vi "merFISH_read_next_task.vi"(3 "error in":errorcluster, 5 "merFISH parameters":T2) -> (0 "error out":errorcluster, 1 "task":T1, 2 "merFISH parameters":T2)   [LabVIEW 2015]
uses:
  CONTROLS/Q_main_element.ctl
  GLOBAL/Global_ABORT.vi
panel:
  out "Instruction":T3(ring)
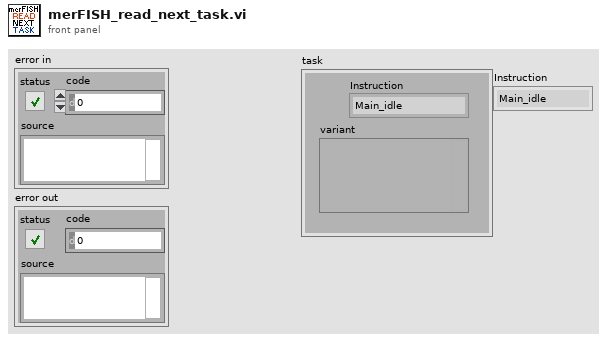
[diagram p1: front panel]
types:
  T1 = typedef "Q_main_element.ctl" = cluster{"variant":variant, "Instruction":enum16{"Main_idle", "Main_initialize", "Main_initialize_TDMS", "Main_initialize_Queue", "Main_error", "Main_DAQ_initialization_results", "Main_ASI_initialization_results", "Main_Piezo_initialization_results", "Main_Valve_initialization_results", "Main_Pump_initialization_results", "Main_CAMERA_initialization_results", "Main_DAQ_error", "Main_ASI_error", "Main_Piezo_error", "Main_CAMERA_error", "Main_Valve_error", "Main_Pump_error", "Main_start_acquiring", "Main_not_acquiring", "Main_acquiring", "Main_stop_acquiring", "Main_change_exposure", "Main_change_z_scan_parameters", "Main_define_ROI", "Main_read_kinetic_time", "Main_cooler", "Main_read_temperature", "Main_save_XY", "Main_load_XY", "Main_discard_XY", "Main_move_to_XY", "Main_measure_QPD", "Main_autofocus_calibration", "Main_save_PID", "Main_change_H_valve_position", "Main_two_way_valve", "Main_save_movie", "Main_init_single_scan", "Main_single_scan", "Main_stop_single_scan", "Main_merFISH_illumination_parameters", "Main_merFISH_buffer_probe_list", "Main_merFISH_injections_procedure", "Main_merFISH_save_setpoint", "Main_merFISH_init", "Main_merFISH_resume", "Main_merFISH_start_autofocus", "Main_merFISH_open_close_valve_merFISH", "Main_merFISH_open_close_valve_photobleaching", "Main_merFISH_hybridization", "Main_merFISH_move_to_ROI", "Main_merFISH_wait_stabilization", "Main_merFISH_scan", "Main_merFISH_photobleaching_injection", "Main_merFISH_photobleaching", "Main_merFISH_save", "Main_merFISH_send_email", "Main_merFISH_close", "Main_TL_define_parameters", "Main_TL_init", "Main_TL_start_autofocus", "Main_TL_move_to_ROI", "Main_TL_wait_for_stabilization", "Main_TL_scan", "Main_TL_wait_cycle_end", "Main_TL_close", "Main_STOP"}}
  T2 = cluster{"XY positions":dbl[][], "Laser lines array":dbl[][], "QPD ref":cluster{"X":dbl, "Y":dbl, "intensity":dbl}, "Ramp":dbl[], "Task list":T1[], "Total # z steps":i32, "merFISH path":path, "merFISH init":cluster{"Autofocus calibrated":bool, "Autofocus setpoint defined":bool, "Laser defined":bool, "ROI defined":bool, "Injection procedure defined":bool}, "Injection procedure IN":i32[][], "merFISH path cluster":cluster{"Z position file path":path, "Acquisition parameters path":path, "Movie path":path}, "Total # frames":i32, "Slope":dbl, "Injection procedure IN photobleaching":i32[][], "Log file":refnum<file>, "Starting time":dbl}
  T3 = enum16{"Main_idle", "Main_initialize", "Main_initialize_TDMS", "Main_initialize_Queue", "Main_error", "Main_DAQ_initialization_results", "Main_ASI_initialization_results", "Main_Piezo_initialization_results", "Main_Valve_initialization_results", "Main_Pump_initialization_results", "Main_CAMERA_initialization_results", "Main_DAQ_error", "Main_ASI_error", "Main_Piezo_error", "Main_CAMERA_error", "Main_Valve_error", "Main_Pump_error", "Main_start_acquiring", "Main_not_acquiring", "Main_acquiring", "Main_stop_acquiring", "Main_change_exposure", "Main_change_z_scan_parameters", "Main_define_ROI", "Main_read_kinetic_time", "Main_cooler", "Main_read_temperature", "Main_save_XY", "Main_load_XY", "Main_discard_XY", "Main_move_to_XY", "Main_measure_QPD", "Main_autofocus_calibration", "Main_save_PID", "Main_change_H_valve_position", "Main_two_way_valve", "Main_save_movie", "Main_init_single_scan", "Main_single_scan", "Main_stop_single_scan", "Main_merFISH_illumination_parameters", "Main_merFISH_buffer_probe_list", "Main_merFISH_injections_procedure", "Main_merFISH_save_setpoint", "Main_merFISH_init", "Main_merFISH_resume", "Main_merFISH_start_autofocus", "Main_merFISH_open_close_valve_merFISH", "Main_merFISH_open_close_valve_photobleaching", "Main_merFISH_hybridization", "Main_merFISH_move_to_ROI", "Main_merFISH_wait_stabilization", "Main_merFISH_scan", "Main_merFISH_photobleaching_injection", "Main_merFISH_photobleaching", "Main_merFISH_save", "Main_merFISH_send_email", "Main_merFISH_close", "Main_TL_define_parameters", "Main_TL_init", "Main_TL_start_autofocus", "Main_TL_move_to_ROI", "Main_TL_wait_for_stabilization", "Main_TL_scan", "Main_TL_wait_cycle_end", "Main_TL_close", "Main_STOP"}
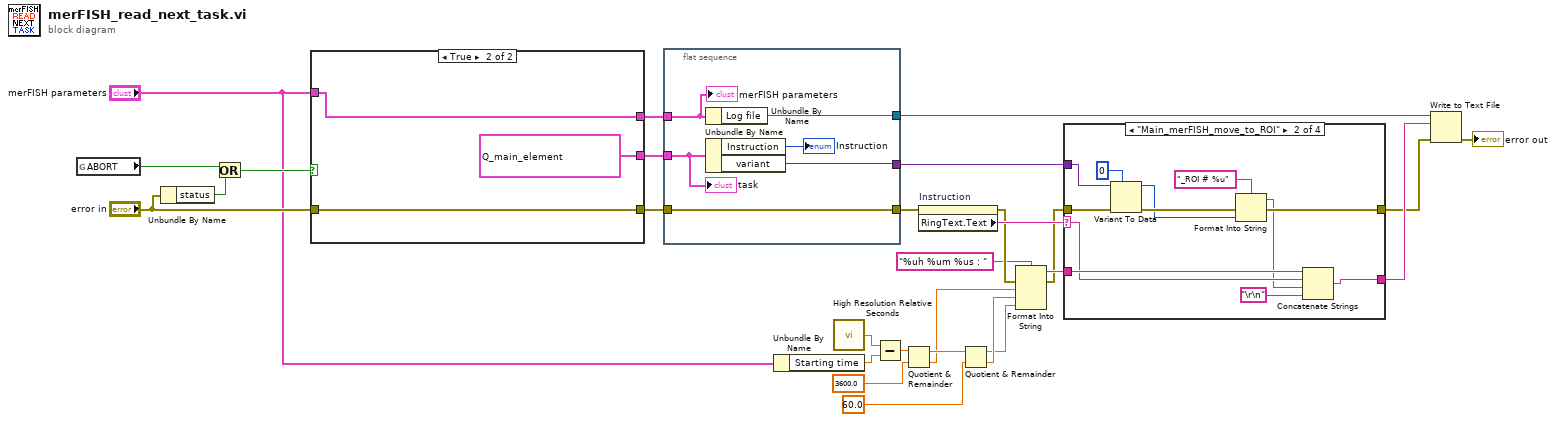
[diagram p0: block diagram]
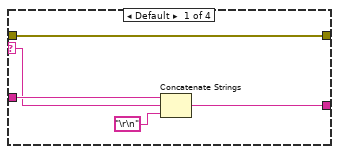
[diagram p2: hidden frame]
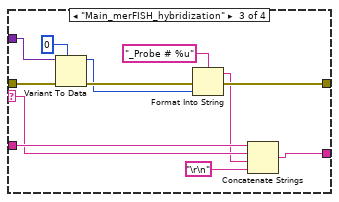
[diagram p3: hidden frame]
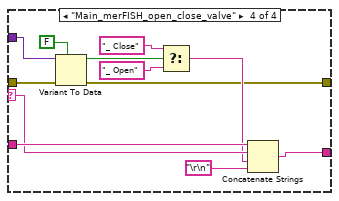
[diagram p4: hidden frame]
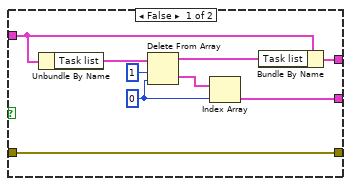
[diagram p5: hidden frame]
diagram:
  n1 = global read "Global_ABORT.vi" "ABORT"() -> (w25:bool)
  n2 = Unbundle By Name("error in") -> ("status"=w26:bool)
  n3 = Or(x=w25, y=w26) -> (x .or. y?=w27:bool)
  n4 = case shown="True" w27 {
    tunnel: [w32 T1 {"variant"=variant, "Instruction"=enum."Main_merFISH_close"} ("element")] -> w23
    tunnel: "merFISH parameters" -> [w31 w39]
    tunnel: [w30 w39] -> w24
    tunnel: "error in" -> [w29 w40]
    tunnel: [w29 w40] -> w20
    frame False {
      w37 = 0 ("index")
      n5 = Unbundle By Name(w31) -> ("Task list"=w34:T1[])
      n6 = Delete From Array(array=w34, length=1, index=w37) -> (deleted portion=w36:T1[], array with subset deleted=w33:T1[])
      n7 = Index Array(array=w36, index=w37) -> (element=w32:T1)
      n8 = Bundle By Name(cluster=w31, "Task list"=w33) -> (w30:T2)
    }
    frame True {
    }
  }
  n9 = flat-sequence {
    tunnel: w24 -> [w41]
    tunnel: w23 -> [w46]
    tunnel: [w44] -> w21
    tunnel: w20 -> [w43]
    tunnel: [w43] -> w19
    tunnel: [w42] -> w16
    frame #0 {
      n10 = Unbundle By Name(w41) -> ("Log file"=w44:refnum<file>)
      n11 = Unbundle By Name(w46) -> ("Instruction"=→"Instruction":T3, "variant"=w42:variant)
      "task" <- w46
      "merFISH parameters" <- w41
    }
  }
  n12 = Unbundle By Name("merFISH parameters") -> ("Starting time"=w12:dbl)
  n13 = call <vilib>:"High Resolution Relative Seconds.vi"() -> ("relative seconds"=w13:dbl)
  n14 = Subtract(x=w13, y=w12) -> (x-y=w11:dbl)
  n15 = Quotient & Remainder(x=w11, y=3600.0) -> (x-y*floor(x/y)=w9:dbl, floor(x/y)=w4:dbl)
  n16 = property on="Instruction" class="Enum (strict)"(error in=w19) -> (error out=w6:errorcluster, "RingText.Text"=w17:string)  [unwired: 1 in, 1 out]
  n17 = Quotient & Remainder(x=w9, y=60.0) -> (x-y*floor(x/y)=w2:dbl, floor(x/y)=w3:dbl)
  n18 = Format Into String(format string="%uh %um %us : " ("initial string"), error in=w6, w4, w3, w2) -> (resulting string=w7:string, error out=w5:errorcluster)  [unwired: 1 in]
  n19 = case shown="\"Main_merFISH_move_to_ROI\"" w17 {
    selector: w17 -> [w49 w59 w71 w84]
    tunnel: w7 -> [w50 w60 w72 w85]
    tunnel: [w48 w53 w65 w82] -> w18
    tunnel: w16 -> [_ w61 w73 w86]
    tunnel: w5 -> [w47 w62 w74 w87]
    tunnel: [w47 w56 w68 w76] -> w15
    frame Default {
      n20 = Concatenate Strings(w50, w49, "\r\n") -> (w48:string)
    }
    frame "Main_merFISH_move_to_ROI" {
      n21 = Variant To Data(error in=w62, type=0 ("x+1"), Variant=w61) -> (data=w57:i32, error out=w58:errorcluster)
      n22 = Format Into String(format string="_ROI # %u" ("string"), error in=w58, w57) -> (resulting string=w55:string, error out=w56:errorcluster)  [unwired: 1 in]
      n23 = Concatenate Strings(w60, w59, w55, "\r\n") -> (w53:string)
    }
    frame "Main_merFISH_hybridization" {
      n24 = Variant To Data(error in=w74, type=0 ("x+1"), Variant=w73) -> (data=w69:i32, error out=w70:errorcluster)
      n25 = Format Into String(format string="_Probe # %u" ("string"), error in=w70, w69) -> (resulting string=w67:string, error out=w68:errorcluster)  [unwired: 1 in]
      n26 = Concatenate Strings(w72, w71, w67, "\r\n") -> (w65:string)
    }
    frame "Main_merFISH_open_close_valve" {
      n27 = Variant To Data(error in=w87, type=FALSE, Variant=w86) -> (data=w77:bool, error out=w76:errorcluster)
      n28 = Select(t="_ Close", s=w77, f="_ Open") -> (s? t:f=w78:string)
      n29 = Concatenate Strings(w85, w84, w78, "\r\n") -> (w82:string)
    }
  }
  n30 = Write to Text File(file (use dialog)=w21, text=w18, error in=w15) -> (error out=→"error out":errorcluster)  [unwired: 1 in, 2 out]
